vi "FIR Windowed Filter Design.vi"() -> ()   [LabVIEW 2010]
uses:
  <vilib>/measure/macond.llb/FIR Filter for 1 Chan.vi
  <vilib>/measure/maspectr.llb/Frequency Response Function (Mag-Phase) 1-1.vi
  <vilib>/Analysis/NI_AALBase.lvlib
  <vilib>/measure/NI_MAPro.lvlib
panel:
  in  "optional FIR filter specification":T1={"PB Gain"=3.0, "SB Gain"=60.0, "Scale"=TRUE, "Window"=enum."None"} {"SB Gain" format="%.2f"; "PB Gain" format="%.2f"}
  in  "FIR filter specifications":T2={"Topology"=enum."Windowed FIR", "Type"=enum."Lowpass", "#Taps"=33, "Lower PB"=100.0, "Upper PB"=30.0, "Lower SB"=200.0, "Upper SB"=0.0} {"Lower SB" format="%.2p"; "Upper SB" format="%.2p"; "Lower PB" format="%.2p"; "Upper PB" format="%.2p"}
  in  "Stop":bool
  in  "view":T3={"dB On (F)"=TRUE, "unwrap phase (F)"=TRUE, "convert to degree (F)"=FALSE}
  out "Phase":cluster{"f0":dbl, "df":dbl, "phase":dbl[]}(graph)={"f0"=0.0, "df"=0.9765625, "phase"=[]}
  out "Magnitude":cluster{"f0":dbl, "df":dbl, "magnitude":dbl[]}(graph)={"f0"=0.0, "df"=0.9765625, "magnitude"=[]}
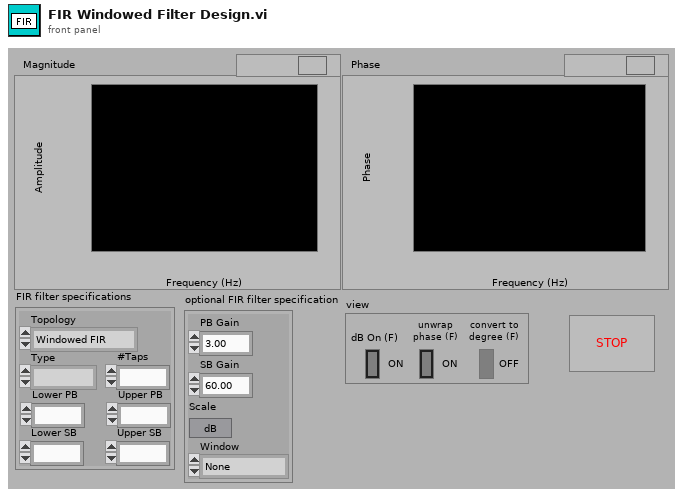
[diagram p1: front panel]
types:
  T1 = cluster{"PB Gain":dbl, "SB Gain":dbl, "Scale":bool, "Window":enum16{"None", "Hanning", "Hamming", "Triangular", "Blackman", "Exact Blackman", "Blackman-Harris", "Kaiser-Bessel", "Flat Top"}}
  T2 = cluster{"Topology":enum16{"Off", "FIR by Specification", "Equi-ripple FIR", "Windowed FIR"}, "Type":enum16{"Lowpass", "Highpass", "Bandpass", "Bandstop"}, "#Taps":i32, "Lower PB":dbl, "Upper PB":dbl, "Lower SB":dbl, "Upper SB":dbl}
  T3 = cluster{"dB On (F)":bool, "unwrap phase (F)":bool, "convert to degree (F)":bool}
  T4 = enum16{"None ", "Hanning", "Hamming", "Blackman-Harris", "Exact Blackman", "Blackman", "Flat Top", "4 Term B-Harris ", "7 Term B-Harris", "Low Sidelobe"}
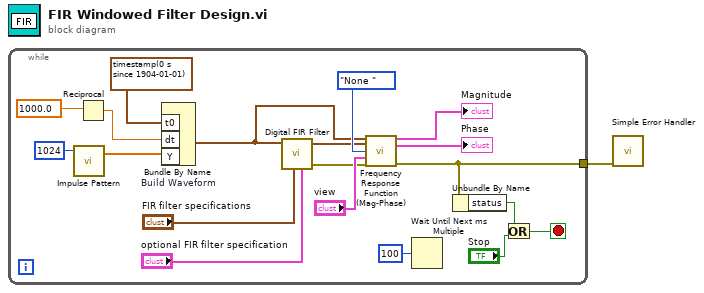
[diagram p0: block diagram]
diagram:
  n1 = while {
    tunnel: [w5] -> w1
    stop <- w2 stop-if-true
    n2 = call <vilib>:"Impulse Pattern.vi"("samples"=1024) -> ("Impulse Pattern"=w14:dbl[])  [unwired: 2 in, 1 out]
    n3 = Reciprocal(x=1000.0) -> (1/x=w18:dbl)
    n4 = Bundle By Name "Build Waveform"("t0"=timestamp(0 s since 1904-01-01), "dt"=w18, "Y"=w14) -> (w12:waveform(dbl))  [unwired: 1 in]
    n5 = call-poly <vilib>:"Digital FIR Filter.vi"("optional FIR filter specifications"="optional FIR filter specification", "FIR filter specifications"="FIR filter specifications", "signal in"=w12) -> ("error out"=w7:errorcluster, "signal out"=w13:waveform(dbl))  [unwired: 6 in, 1 out]
    n6 = call-poly <vilib>:"Frequency Response Function (Mag-Phase).vi"("time signal X"=w12, "time signal Y"=w13, "window"=T4."None ", "view"="view", "error in (no error)"=w7) -> ("magnitude"=→"Magnitude":cluster{"f0":dbl, "df":dbl, "magnitude":dbl[]}, "phase"=→"Phase":cluster{"f0":dbl, "df":dbl, "phase":dbl[]}, "error out"=w5:errorcluster)  [unwired: 5 in, 3 out]
    n7 = Wait Until Next ms Multiple(millisecond multiple=u32 100) -> ()  [unwired: 1 out]
    n8 = Unbundle By Name "Unbundle By Name"(w5) -> ("status"=w4:bool)
    n9 = Or(x=w4, y="Stop") -> (x .or. y?=w2:bool)
  }
  n10 = call <vilib>:"Simple Error Handler.vi"("error in (no error)"=w1) -> ()  [unwired: 4 in, 5 out]
